vi "readSignalFile.vi"(2 "Путь к записи сигнала":path=path "C:/Users/ira_1/OneDrive/Рабочий стол/samples.bin", 3 "Целое число строк записанного файла":i32=100) -> (0 "Array 2":cdb[][](array[numeric]), 1 "subarray":cdb[](array[numeric]))   [LabVIEW 2020]
panel:
  out "Array 3":cdb[](array[numeric])
  out "size(s)":i32[](array[numeric])
  out "Array":dbl[][](array[numeric])
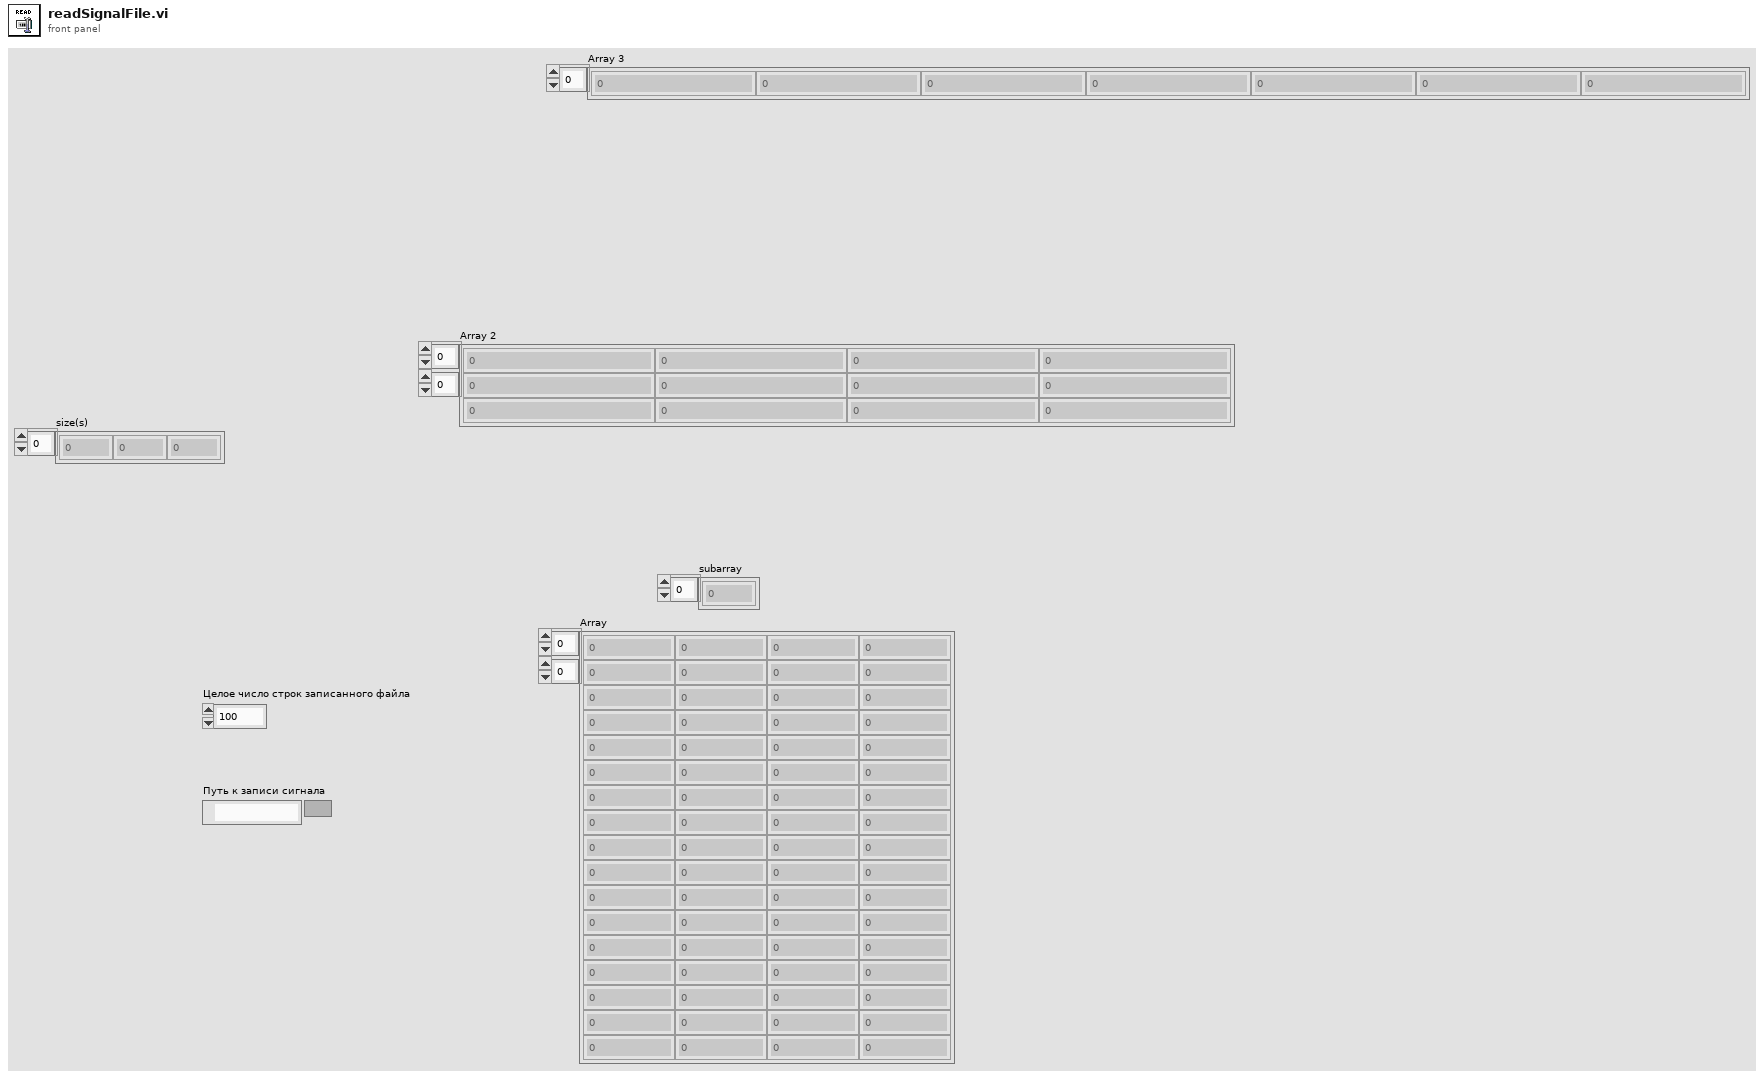
[diagram p1: front panel]
types:
  T1 = enum16{"open", "replace", "create", "open or create", "replace or create", "replace or create with confirmation"}
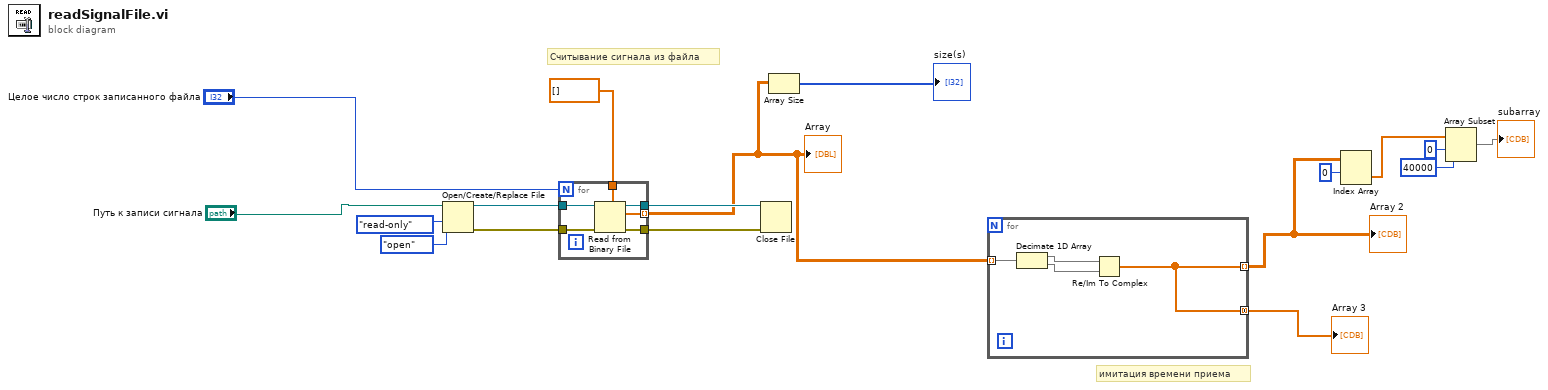
[diagram p0: block diagram]
diagram:
  # "имитация времени приема"
  # "Считывание сигнала из файла"
  n1 = Open/Create/Replace File(file path (use dialog)="Путь к записи сигнала", operation (0:open)=T1."open", access (0:read/write)=enum16{"read/write", "read-only", "write-only"}."read-only") -> (refnum out=w18:refnum<file>, error out=w17:errorcluster)  [unwired: 3 in, 1 out]
  n2 = for {
    N: "Целое число строк записанного файла" -> [_]
    tunnel: w18 -> [w24]
    tunnel: w17 -> [w23]
    tunnel: dbl[] [] -> [w22]
    tunnel: [w21] -> w9 mode=indexing
    tunnel: [w20] -> w13
    tunnel: [w19] -> w12
    n3 = Read from Binary File(5:w22, 8:w23, 11:w24) -> (0:w19:errorcluster, 2:w21:dbl[], 3:w20:refnum<file>)  [unwired: 3 in, 1 out]
  }
  "Array" <- w9
  n4 = Close File(refnum=w13, error in=w12) -> ()  [unwired: 2 out]
  n5 = Array Size(array=w9) -> (size(s)=→"size(s)":i32[])
  n6 = for {
    tunnel: w9 -> [w28] mode=indexing
    tunnel: [w25] -> w6 mode=indexing
    tunnel: [w25] -> w7 mode=concatenating
    n7 = Decimate 1D Array(w28) -> (w27:dbl[], w26:dbl[])
    n8 = Re/Im To Complex(1:w26, 2:w27) -> (0:w25:cdb[])
  }
  "Array 2" <- w6
  "Array 3" <- w7
  n9 = Index Array(array=w6, index (row)=0) -> (element=w4:cdb[])  [unwired: 1 in]
  n10 = Array Subset(array=w4, index=0, length=40000) -> (→"subarray":cdb[])
